vi "App.vi"() -> ()   [LabVIEW 2023]
uses:
  LabView_IoT_Termopar-main/Customized_Control_ON_OFF.ctl
  <vilib>/Instr/_visa.llb/VISA Configure Serial Port (Instr).vi
  <vilib>/httpClient/POSTBuffer.vi
  <vilib>/httpClient/LabVIEWHTTPClient.lvlib
panel:
  out "Valor":dbl=30.25
  in  "Tasa de Muestreo":dbl=1030.0
  in  "Inicio":T1
  out "Estado":bool
  in  "STOP":bool
  out "Señal":dbl(graph)=30.25
  in  "Puerto de comunicación":refnum<visa-resource-name>="COM3"
  # "MEDICIÓN DE TEMPERATURA"
  # "UNIVERSIDAD NACIONAL AUTÓNOMA DE MÉXICO"
  # "INSTRUMENTACIÓN VIRTUAL"
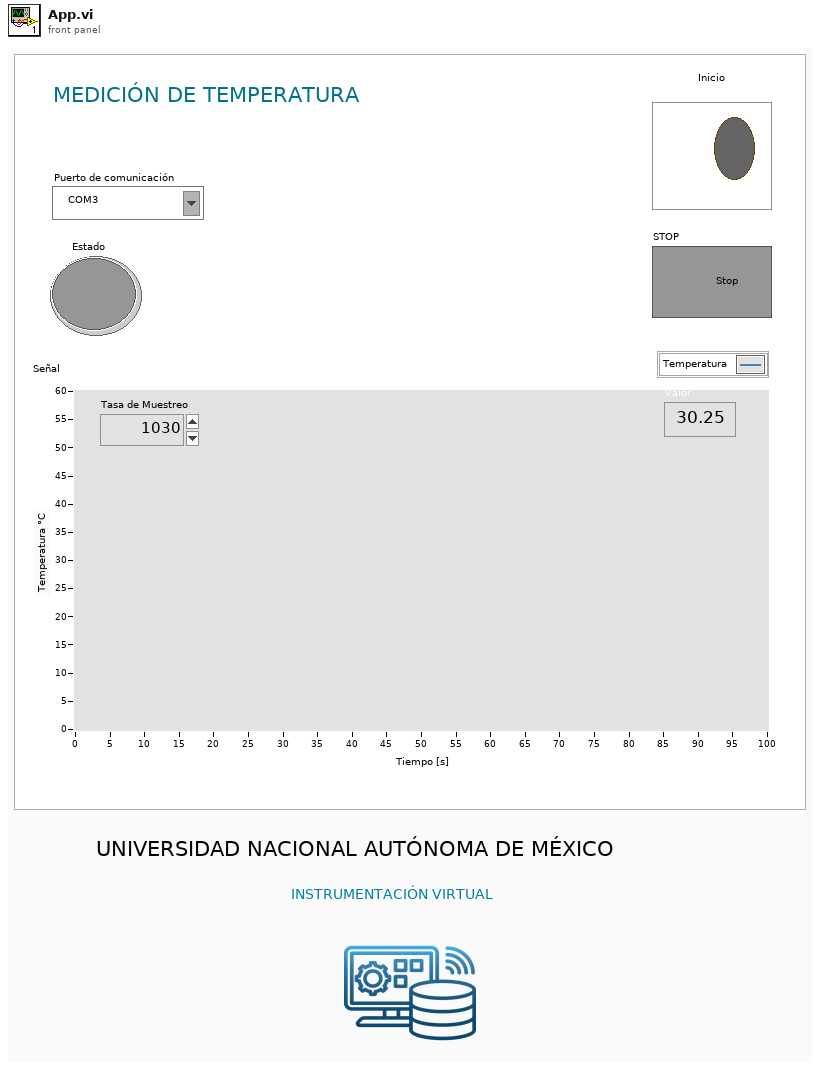
[diagram p1: front panel]
types:
  T1 = typedef "Customized_Control_ON_OFF.ctl" = bool
  T2 = typedef "LabVIEWHTTPClient.lvlib/ClientHandle.ctl" = refnum<k1>
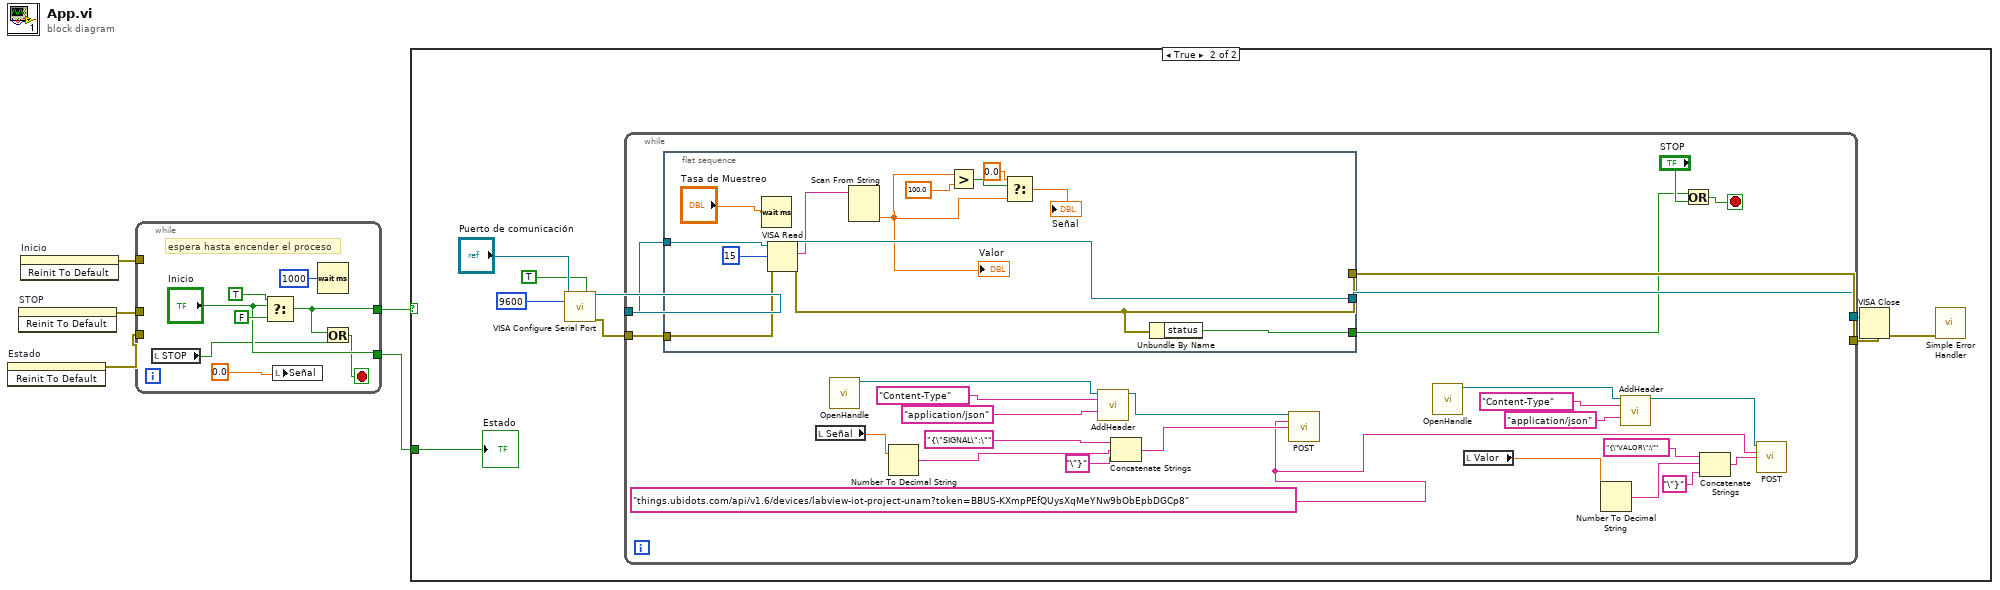
[diagram p0: block diagram]
diagram:
  n1 = invoke on="Estado" class="Bool (strict)" method="Reinit To Default"() -> (error out=w1:errorcluster)  [unwired: 3 in, 2 out]
  n2 = invoke on="STOP" class="Bool (strict)" method="Reinit To Default"() -> (error out=w3:errorcluster)  [unwired: 3 in, 2 out]
  n3 = invoke on="Inicio" class="Bool (strict)" method="Reinit To Default"() -> (error out=w2:errorcluster)  [unwired: 3 in, 2 out]
  n4 = while {
    tunnel: [w8] -> w5
    tunnel: ["Inicio"] -> w4
    tunnel: w3 -> [_]
    tunnel: w2 -> [_]
    tunnel: w1 -> [_]
    stop <- w6 stop-if-true
    # "espera hasta encender el proceso"
    n5 = local read "STOP"() -> (w7:bool)
    n6 = Select(t=TRUE, s="Inicio", f=FALSE) -> (s? t:f=w8:bool)
    n7 = local write "Señal"(0.0 ("Señal")) -> ()
    n8 = Wait (ms)(milliseconds to wait=u32 1000) -> ()  [unwired: 1 out]
    n9 = Or(x=w8, y=w7) -> (x .or. y?=w6:bool)
  }
  n10 = case shown="True" w5 {
    tunnel: w4 -> [_ w14]
    frame False {
    }
    frame True {
      n11 = call-poly "VISA Configure Serial Port"("VISA resource name"="Puerto de comunicación", "Enable Termination\nChar (T)"=TRUE ("Enable Termination\nChar (T)"), "baud rate (9600)"=u32 9600) -> ("VISA resource name out"=w19:refnum<visa-resource-name>, "error out"=w18:errorcluster)  [unwired: 11 in]
      n12 = while {
        tunnel: w19 -> [w28]
        tunnel: w18 -> [w29]
        tunnel: [w26] -> w16
        tunnel: [w27] -> w15
        stop <- w48 stop-if-true
        w38 = "things.ubidots.com/api/v1.6/devices/labview-iot-project-unam?token=BBUS-KXmpPEfQUysXqMeYNw9bObEpbDGCp8"
        n13 = flat-sequence {
          tunnel: [w59] -> w25
          tunnel: [w60] -> w26
          tunnel: [w61] -> w27
          tunnel: w28 -> [w56]
          tunnel: w29 -> [w58]
          frame #0 {
            n14 = Wait (ms)(milliseconds to wait="Tasa de Muestreo") -> ()  [unwired: 1 out]
            n15 = VISA Read(VISA resource name=w56, byte count=u32 15, error in (no error)=w58) -> (VISA resource name out=w60:refnum<visa-resource-name>, read buffer=w55:string, error out=w61:errorcluster)  [unwired: 1 out]
            n16 = Scan From String(input string=w55) -> (output 1=w49:dbl)  [unwired: 4 in, 3 out]
            "Valor" <- w49
            n17 = Greater?(x=w49, y=100.0) -> (0:w51:bool)
            n18 = Select(t=0.0, s=w51, f=w49) -> (s? t:f=→"Señal":dbl)
            n19 = Unbundle By Name(w61) -> ("status"=w59:bool)
          }
        }
        n20 = local read "Señal"() -> (w42:dbl)
        n21 = call <vilib>:"OpenHandle.vi"() -> ("client handle out"=w34:T2)  [unwired: 14 in, 1 out]
        n22 = Number To Decimal String(number=w42) -> (decimal integer string=w43:string)  [unwired: 1 in]
        n23 = call <vilib>:"AddHeader.vi"("client handle"=w34, "header"="Content-Type", "value"="application/json") -> ("client handle out"=w37:T2)  [unwired: 11 in, 1 out]
        n24 = Concatenate Strings("{\"SIGNAL\":\"" ("string"), w43, "\"}" ("string")) -> (w44:string)
        n25 = call-poly <vilib>:"POST.vi"("client handle"=w37, "url"=w38, "buffer"=w44) -> ()  [unwired: 9 in, 4 out]
        n26 = call <vilib>:"OpenHandle.vi"() -> ("client handle out"=w33:T2)  [unwired: 14 in, 1 out]
        n27 = local read "Valor"() -> (w24:dbl)
        n28 = Number To Decimal String(number=w24) -> (decimal integer string=w23:string)  [unwired: 1 in]
        n29 = call <vilib>:"AddHeader.vi"("client handle"=w33, "header"="Content-Type", "value"="application/json") -> ("client handle out"=w30:T2)  [unwired: 11 in, 1 out]
        n30 = Or(x=w25, y="STOP") -> (x .or. y?=w48:bool)
        n31 = Concatenate Strings("{\"VALOR\":\"" ("string"), w23, "\"}" ("string")) -> (w39:string)
        n32 = call-poly <vilib>:"POST.vi"("client handle"=w30, "url"=w38, "buffer"=w39) -> ()  [unwired: 9 in, 4 out]
      }
      n33 = VISA Close(VISA resource name=w16, error in (no error)=w15) -> (error out=w17:errorcluster)
      n34 = call <vilib>:"Simple Error Handler.vi"("error in (no error)"=w17) -> ()  [unwired: 4 in, 5 out]
      "Estado" <- w14
    }
  }
